vi "SAOMM-UpdateROI.vi"(0 "PRAMMS-COMM IN":refnum<visa-resource-name>="COM4", 1 "Active Refnum":refnum<vi>, 2 "PrAMS-ACK":refnum<vi>, 3 "MessageType":cluster{string[], u32[]}, 11 "Error IN":errorcluster, 12 "Position":cluster{"Offset Y":u16, "Offset X":u16}) -> (4 "PRAMMS-COMM OUT":refnum<visa-resource-name>="COM4", 8 "Error":bool, 15 "Error OUT":errorcluster)   [LabVIEW 2019]
uses:
  Polymorphics/Num2littleEndian(U16).vi
panel:
  in  "Signature":u32=1886544237
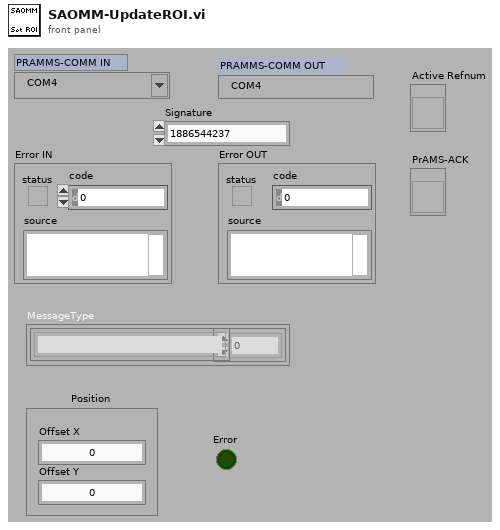
[diagram p1: front panel]
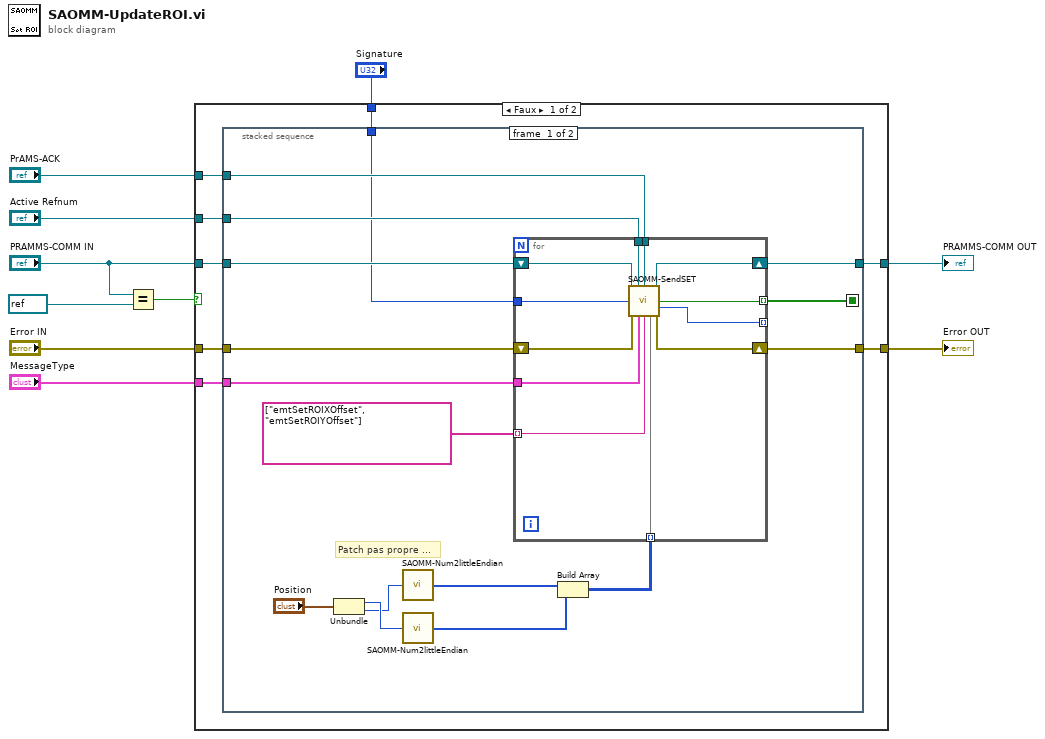
[diagram p0: block diagram]
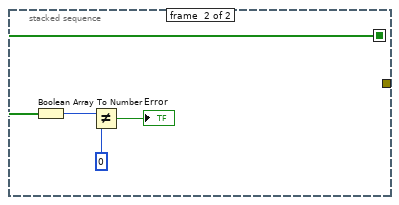
[diagram p2: hidden frame]
diagram:
  n1 = Equal?(x="PRAMMS-COMM IN", y=refnum<visa-resource-name> "-1") -> (x = y?=w9:bool)
  n2 = case shown="Faux" w9 {
    tunnel: "PRAMMS-COMM IN" -> [w18 w52]
    tunnel: "Error IN" -> [w17 w51]
    tunnel: [w16 w52] -> w6
    tunnel: [w15 w51] -> w5
    tunnel: "Active Refnum" -> [w14 _]
    tunnel: "PrAMS-ACK" -> [w13 _]
    tunnel: "Signature" -> [w12 _]
    tunnel: "MessageType" -> [w11 _]
    frame False {
      n3 = stacked-sequence {
        seq-local: [w24 _] -> [_ w47]
        tunnel: w18 -> [w33 _]
        tunnel: w17 -> [w32 _]
        tunnel: [w22 _] -> w16
        tunnel: [w21 _] -> w15
        tunnel: w14 -> [w27 _]
        tunnel: w13 -> [w26 _]
        tunnel: w12 -> [w25 _]
        tunnel: w11 -> [w23 _]
        frame #0 {
          # "Patch pas propre ..."
          n4 = Unbundle("Position") -> ("Offset Y"=w20:u16, "Offset X"=w19:u16)
          n5 = call-poly "SAOMM-Num2littleEndian.vi"("Number"=w19) -> ("LiitleEndianedData"=w30:u8[])  [unwired: 14 in]
          n6 = call-poly "SAOMM-Num2littleEndian.vi"("Number"=w20) -> ("LiitleEndianedData"=w29:u8[])  [unwired: 14 in]
          n7 = Build Array(w30, w29) -> (w34:u8[][])
          n8 = for {
            tunnel: w34 -> [w39] mode=indexing
            shift-right: [w44] -> w22
            shift-left: w33 -> [w45]
            shift-right: [w43] -> w21
            shift-left: w32 -> [w46]
            tunnel: string[] ["emtSetROIXOffset", "emtSetROIYOffset"] -> [w40] mode=indexing
            tunnel: w26 -> [w41]
            tunnel: w27 -> [w42]
            tunnel: [w38] -> w24 mode=indexing
            tunnel: w23 -> [w37]
            tunnel: w25 -> [w36]
            tunnel: [w35] -> _ mode=indexing
            n9 = call "SAOMM-SendSET.vi"("PRAMMS-COMM IN"=w45, "Active Refnum"=w42, "PrAMS-ACK"=w41, "Signature"=w36, "Error IN"=w46, "MessageType"=w37, "Active SET"=w40, "Value (little endianed byte array)"=w39) -> ("PRAMMS-COMM OUT"=w44:refnum<visa-resource-name>, "Error"=w38:bool, "WaitACKTime"=w35:u32, "Error OUT"=w43:errorcluster)  [unwired: 4 in]
          }
        }
        frame #1 {
          n10 = Boolean Array To Number(Boolean array=w47) -> (number=w50:u32)
          n11 = Not Equal?(x=w50, y=u32 0) -> (x != y?=→"Error":bool)
        }
      }
    }
    frame True {
    }
  }
  "Error OUT" <- w5
  "PRAMMS-COMM OUT" <- w6
